vi "BP Save.vi"(8 "error in":errorcluster, 10 "View Model in":T1, 11 "TDMS in":refnum<class "TDMS.lvclass">) -> (0 "error out":errorcluster, 3 "TDMS out":refnum<class "TDMS.lvclass">)   [LabVIEW 2017, in "Report_lib.lvlib" / "TDMS.lvclass"]
uses:
  TDMS.lvclass
  View Model/Controls/View Model.ctl
  View Model/Controls/Shared Model.ctl
  Error Handler/Controls/Error Model.ctl
  Error Handler/Controls/Error Event.ctl
  Error Handler/Controls/Error Type.ctl
  Controller/Controls/Controller Model.ctl
  Controller/Controls/Controller Event.ctl
  Controller/Controls/Controller Command.ctl
  Controller/Controls/Controller Overhead.ctl
  Real-Time/RT Status.ctl
  Real-Time/RT Loop Status.ctl
  Controller/Controls/Controller NStream.ctl
  Controller/Controls/Controller DAQ Data.ctl
  TDMS Logger/Controls/TDMS Model.ctl
  TDMS Logger/Controls/TDMS Event.ctl
  TDMS Logger/Controls/TDMS Command.ctl
  TDMS Logger/Controls/TDMS Overhead.ctl
  TDMS Logger/Controls/TDMS ChanProperties.ctl
  TDMS.lvclass/TDMS.ctl
panel:
  out "DIM":i32
  out "size(s)":i32
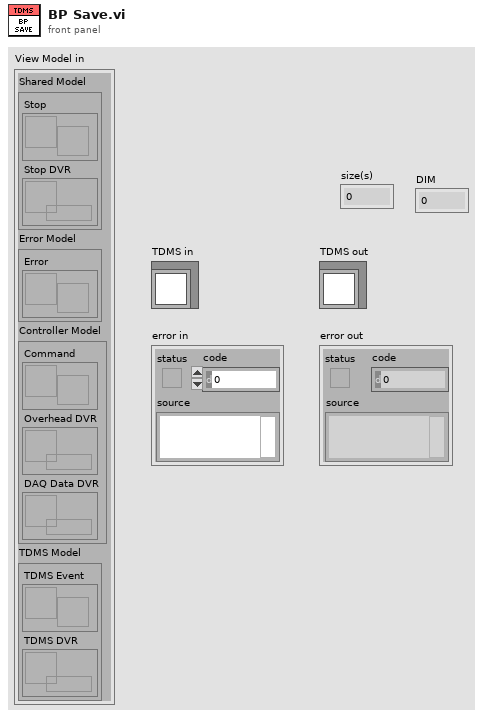
[diagram p1: front panel]
types:
  T1 = typedef "View Model.ctl" = cluster{"Shared Model":T2, "Error Model":T3, "Controller Model":T4, "TDMS Model":T5}
  T2 = typedef "Shared Model.ctl" = cluster{"Stop":refnum<user-event>, "Stop DVR":refnum<data-value>}
  T3 = typedef "Error Model.ctl" = cluster{"Error":refnum<user-event>}
  T4 = typedef "Controller Model.ctl" = cluster{"Command":refnum<user-event>, "Overhead DVR":refnum<data-value>, "DAQ Data DVR":refnum<data-value>}
  T5 = typedef "TDMS Model.ctl" = cluster{"TDMS Event":refnum<user-event>, "TDMS DVR":refnum<data-value>}
  T6 = typedef "TDMS ChanProperties.ctl" = cluster{"AOM9":string[][], "AIM2":string[][], "DIM3":string[][], "DIM4":string[][], "DOM6":string[][], "DOM7":string[][]}
  T7 = typedef "Controller DAQ Data.ctl" = cluster{"AOM data":dbl[], "AIMV data":dbl[], "AIMC data":dbl[], "DOM data":dbl[], "DIM data":dbl[], "AOM timestamp":dbl, "AIMV timestamp":dbl, "AIMC timestamp":dbl, "DOM timestamp":dbl, "DIM timestamp":dbl}
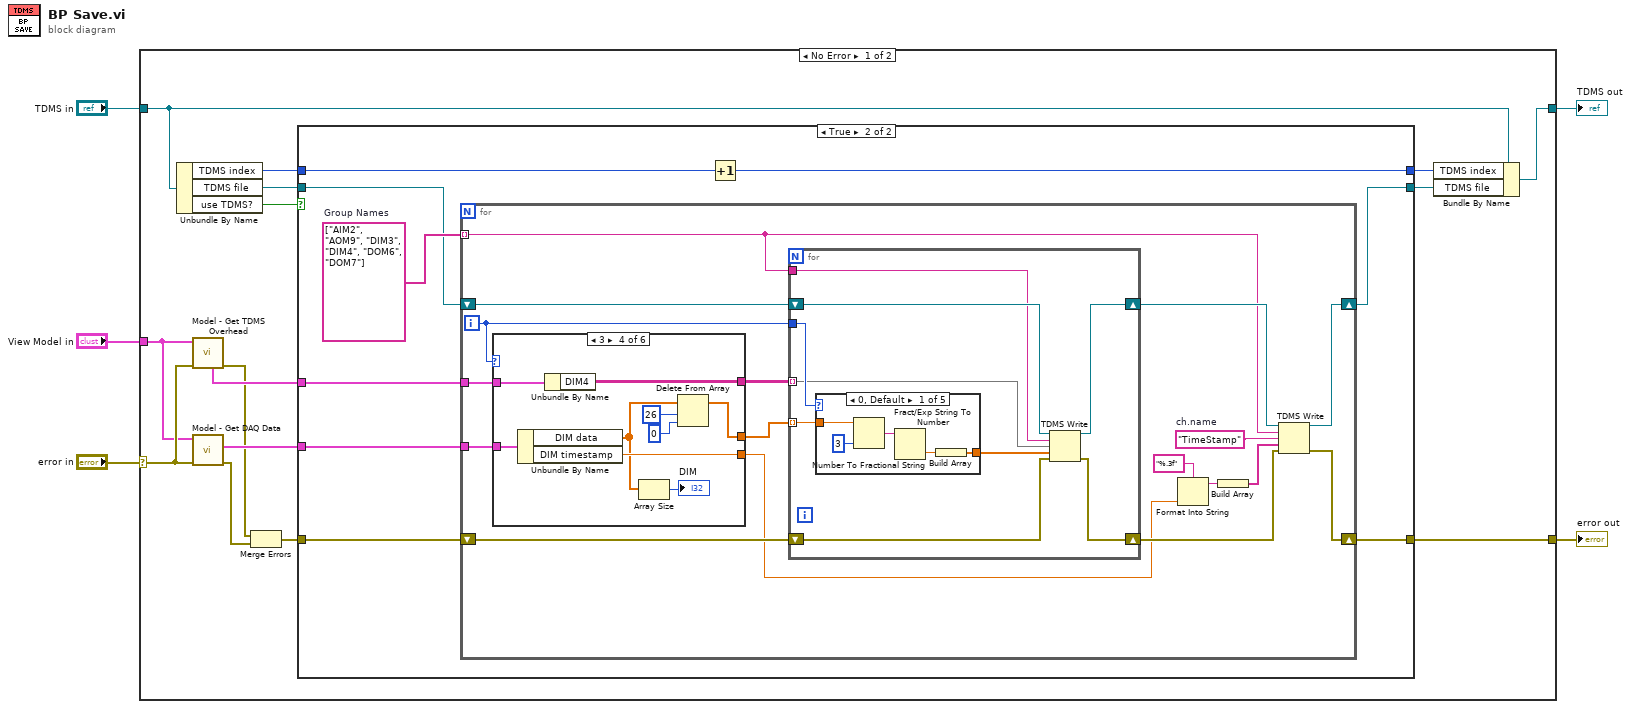
[diagram p0: block diagram]
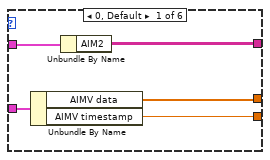
[diagram p3: hidden frame]
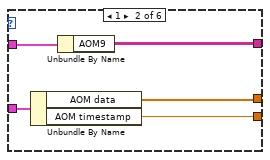
[diagram p4: hidden frame]
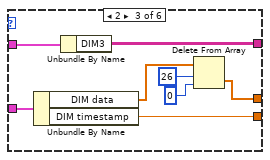
[diagram p5: hidden frame]
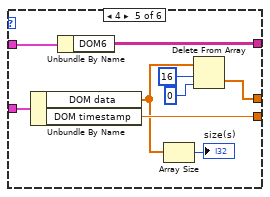
[diagram p6: hidden frame]
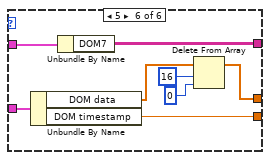
[diagram p7: hidden frame]
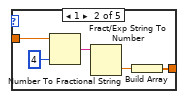
[diagram p8: hidden frame]
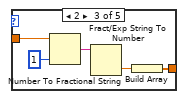
[diagram p9: hidden frame]
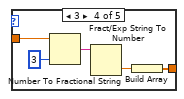
[diagram p10: hidden frame]
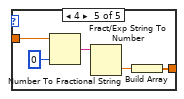
[diagram p11: hidden frame]
diagram:
  n1 = case shown="No Error" "error in" {
    selector: "error in" -> [w11 w129]
    tunnel: [w14 w129] -> w2
    tunnel: [w15 w128] -> w3
    tunnel: "TDMS in" -> [w16 w128]
    tunnel: "View Model in" -> [w10 _]
    frame No Error {
      n2 = Unbundle By Name(w16) -> ("TDMS index"=w19:i32, "TDMS file"=w20:refnum<k34>, "use TDMS?"=w13:bool)
      n3 = call "Model - Get TDMS Overhead.vi"("error in (no error)"=w11, "View Model"=w10) -> ("error out"=w7:errorcluster, "ChProps"=w12:T6)  [unwired: 4 in, 4 out]
      n4 = call "Model - Get DAQ Data.vi"("error in (no error)"=w11, "View Model"=w10) -> ("error out"=w8:errorcluster, "DAQ Data"=w9:T7)  [unwired: 7 in, 1 out]
      n5 = Merge Errors(w7, w8) -> (w6:errorcluster)
      n6 = case shown="True" w13 {
        tunnel: w20 -> [w22 w31]
        tunnel: w6 -> [w21 w30]
        tunnel: w19 -> [w23 w29]
        tunnel: [w23 w28] -> w18
        tunnel: [w22 w27] -> w17
        tunnel: w9 -> [_ w26]
        tunnel: [w21 w25] -> w14
        tunnel: w12 -> [_ w24]
        frame False {
        }
        frame True {
          w32 = string[] ["AIM2", "AOM9", "DIM3", "DIM4", "DOM6", "DOM7"]  # Group Names
          n7 = for {
            tunnel: w32 -> [w35] mode=indexing
            tunnel: w24 -> [w48]
            tunnel: w26 -> [w49]
            shift-right: [w34] -> w27
            shift-left: w31 -> [w44]
            shift-right: [w33] -> w25
            shift-left: w30 -> [w43]
            i -> [w45]
            w42 = "TimeStamp"  # ch.name
            n8 = case shown="3" w45 {
              tunnel: w49 -> [w54 w59 w67 w76 w85 w93]
              tunnel: w48 -> [w53 w58 w66 w75 w84 w92]
              tunnel: [w52 w57 w61 w70 w79 w86] -> w47
              tunnel: [w51 w56 w65 w74 w83 w91] -> w46
              tunnel: [w50 w55 w64 w73 w82 w90] -> w37
              frame 0, Default {
                n9 = Unbundle By Name(w54) -> ("AIMV data"=w52:dbl[], "AIMV timestamp"=w50:dbl)
                n10 = Unbundle By Name(w53) -> ("AIM2"=w51:string[][])
              }
              frame 1 {
                n11 = Unbundle By Name(w59) -> ("AOM data"=w57:dbl[], "AOM timestamp"=w55:dbl)
                n12 = Unbundle By Name(w58) -> ("AOM9"=w56:string[][])
              }
              frame 2 {
                n13 = Unbundle By Name(w67) -> ("DIM data"=w60:dbl[], "DIM timestamp"=w64:dbl)
                n14 = Unbundle By Name(w66) -> ("DIM3"=w65:string[][])
                n15 = Delete From Array(array=w60, length=26, index=0) -> (deleted portion=w61:dbl[])  [unwired: 1 out]
              }
              frame 3 {
                n16 = Unbundle By Name(w76) -> ("DIM data"=w68:dbl[], "DIM timestamp"=w73:dbl)
                n17 = Unbundle By Name(w75) -> ("DIM4"=w74:string[][])
                n18 = Array Size(array=w68) -> (size(s)=→"DIM":i32)
                n19 = Delete From Array(array=w68, length=26, index=0) -> (array with subset deleted=w70:dbl[])  [unwired: 1 out]
              }
              frame 4 {
                n20 = Unbundle By Name(w85) -> ("DOM data"=w77:dbl[], "DOM timestamp"=w82:dbl)
                n21 = Unbundle By Name(w84) -> ("DOM6"=w83:string[][])
                n22 = Array Size(array=w77) -> (size(s)=→"size(s)":i32)
                n23 = Delete From Array(array=w77, length=16, index=0) -> (deleted portion=w79:dbl[])  [unwired: 1 out]
              }
              frame 5 {
                n24 = Unbundle By Name(w93) -> ("DOM data"=w89:dbl[], "DOM timestamp"=w90:dbl)
                n25 = Unbundle By Name(w92) -> ("DOM7"=w91:string[][])
                n26 = Delete From Array(array=w89, length=16, index=0) -> (array with subset deleted=w86:dbl[])  [unwired: 1 out]
              }
            }
            n27 = for {
              tunnel: w47 -> [w101] mode=indexing
              tunnel: w46 -> [w98] mode=indexing
              tunnel: w45 -> [w102]
              shift-right: [w99] -> w39
              shift-left: w44 -> [w100]
              tunnel: w35 -> [w97]
              shift-right: [w94] -> w40
              shift-left: w43 -> [w95]
              n28 = case shown="0, Default" w102 {
                tunnel: w101 -> [w104 w109 w114 w119 w124]
                tunnel: [w103 w108 w113 w118 w123] -> w96
                frame 0, Default {
                  n29 = Number To Fractional String(number=w104, precision (6)=i16 3) -> (F-format string=w106:string)  [unwired: 2 in]
                  n30 = Fract/Exp String To Number(string=w106) -> (number=w107:dbl)  [unwired: 3 in, 1 out]
                  n31 = Build Array(w107) -> (w103:dbl[])
                }
                frame 1 {
                  n32 = Number To Fractional String(number=w109, precision (6)=i16 4) -> (F-format string=w111:string)  [unwired: 2 in]
                  n33 = Fract/Exp String To Number(string=w111) -> (number=w112:dbl)  [unwired: 3 in, 1 out]
                  n34 = Build Array(w112) -> (w108:dbl[])
                }
                frame 2 {
                  n35 = Number To Fractional String(number=w114, precision (6)=i16 1) -> (F-format string=w116:string)  [unwired: 2 in]
                  n36 = Fract/Exp String To Number(string=w116) -> (number=w117:dbl)  [unwired: 3 in, 1 out]
                  n37 = Build Array(w117) -> (w113:dbl[])
                }
                frame 3 {
                  n38 = Number To Fractional String(number=w119, precision (6)=i16 3) -> (F-format string=w121:string)  [unwired: 2 in]
                  n39 = Fract/Exp String To Number(string=w121) -> (number=w122:dbl)  [unwired: 3 in, 1 out]
                  n40 = Build Array(w122) -> (w118:dbl[])
                }
                frame 4 {
                  n41 = Number To Fractional String(number=w124, precision (6)=i16 0) -> (F-format string=w126:string)  [unwired: 2 in]
                  n42 = Fract/Exp String To Number(string=w126) -> (number=w127:dbl)  [unwired: 3 in, 1 out]
                  n43 = Build Array(w127) -> (w123:dbl[])
                }
              }
              n44 = TDMS Write(0:w100, 5:w97, 7:w98, 9:w96, 11:w95) -> (4:w99:refnum<k34>, 15:w94:errorcluster)  [unwired: 1 in, 2 out]
            }
            n45 = Format Into String(format string="%.3f", w37) -> (resulting string=w36:string)  [unwired: 2 in, 1 out]
            n46 = Build Array(w36) -> (w41:string[])
            n47 = TDMS Write(0:w39, 5:w35, 7:w42, 9:w41, 11:w40) -> (4:w34:refnum<k34>, 15:w33:errorcluster)  [unwired: 1 in, 2 out]
          }
          n48 = Increment(x=w29) -> (x+1=w28:i32)
        }
      }
      n49 = Bundle By Name(cluster=w16, "TDMS index"=w18, "TDMS file"=w17) -> (w15:refnum<class "TDMS.lvclass">)
    }
    frame Error {
    }
  }
  "error out" <- w2
  "TDMS out" <- w3
